vi "REPORT SHOW.vi"(10 "report Path":path) -> (2 "true":bool)   [LabVIEW 2018]
panel:
  in  "error in (no error)":errorcluster caption="错误输入（无错误）"
  out "error out":errorcluster caption="错误输出"
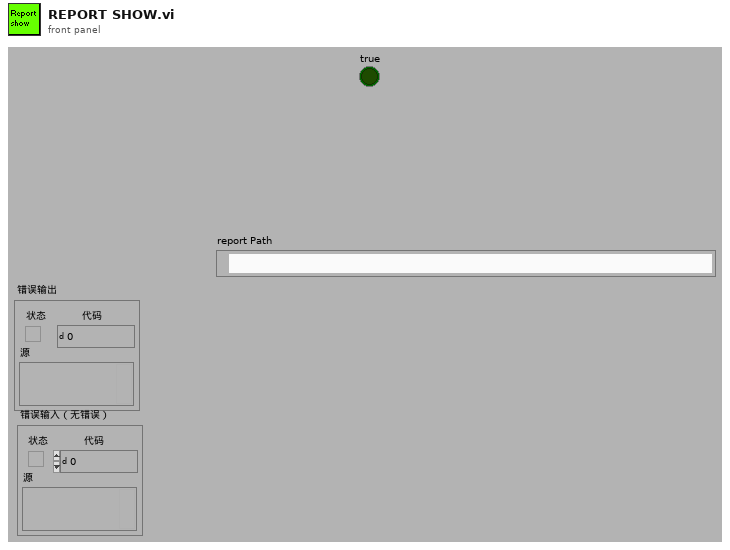
[diagram p1: front panel]
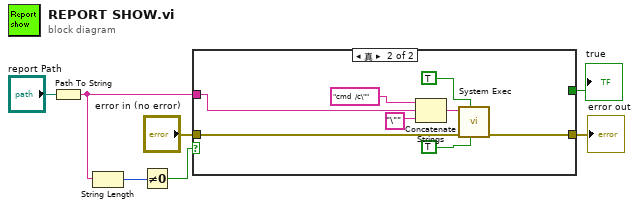
[diagram p0: block diagram]
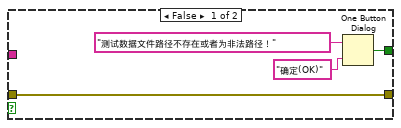
[diagram p2: hidden frame]
diagram:
  n1 = Path To String(path="report Path") -> (string=w5:string)
  n2 = String Length(string=w5) -> (length=w4:i32)
  n3 = Not Equal To 0?(x=w4) -> (x != 0?=w3:bool)
  n4 = case shown="真" w3 {
    tunnel: [w9 w19] -> w6
    tunnel: "error in (no error)" -> [w9 w18]
    tunnel: w5 -> [_ w17]
    tunnel: [w8 _] -> w1
    frame False {
      n5 = One Button Dialog(message="测试数据文件路径不存在或者为非法路径！" ("消息"), button name ("OK")="确定(OK)" ("按钮名称（“确定”）")) -> (true=w8:bool)
    }
    frame True {
      n6 = Concatenate Strings("cmd  /c\"" ("command line"), w17, "\"") -> (w14:string)
      n7 = call <vilib>:"System Exec.vi"("run minimized? (F)"=TRUE, "wait until completion? (T)"=TRUE, "error in (no error)"=w18, "command line"=w14) -> ("error out"=w19:errorcluster)  [unwired: 2 in, 5 out]
    }
  }
  "error out" <- w6
  "true" <- w1
